vi "User Stop Event.vi"(0 "Stop":T2, 11 "Error in":errorcluster, 13 "Operations":T1) -> (4 "Stop Ref":refnum<user-event>, 15 "Error out":errorcluster)   [LabVIEW 2020, in "Data Communication Receiver.lvlib"]
doc: "User Event LV2 to stop the producer of the receiver."
uses:
  Data Communication Receiver.lvlib
  Typedefs/User Event Stop Data.ctl
  Typedefs/User event Operations.ctl
  Transmitter/Data Communication Transmitter.lvlib
panel:
  # "USER EVENT"
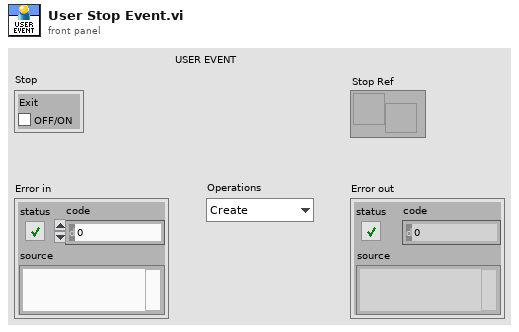
[diagram p1: front panel]
types:
  T1 = typedef "Data Communication Transmitter.lvlib/User event Operations.ctl" = enum16{"Create", "Generate", "Get Ref", "destroy"}
  T2 = typedef "Data Communication Receiver.lvlib/User Event Stop Data.ctl" = cluster{"Exit":bool}
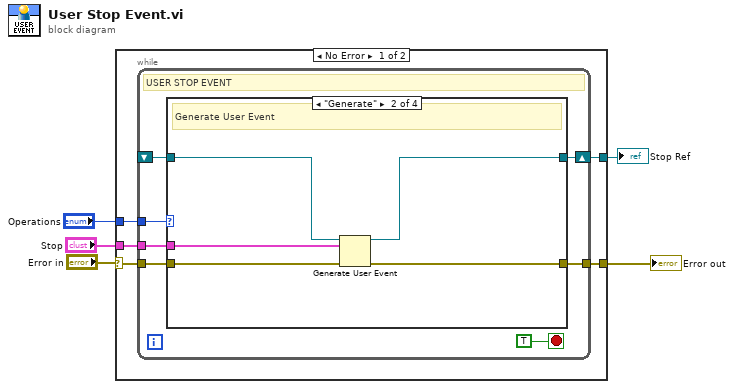
[diagram p0: block diagram]
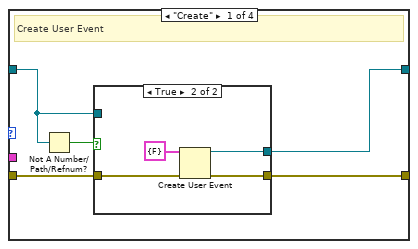
[diagram p2: hidden frame]
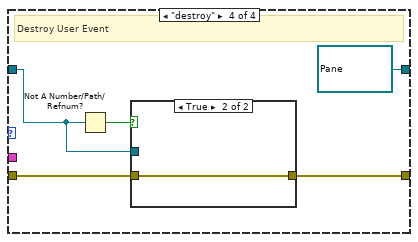
[diagram p5: hidden frame]
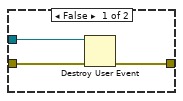
[diagram p6: hidden frame]
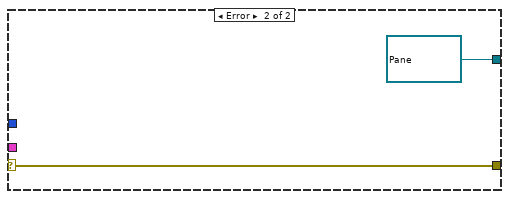
[diagram p7: hidden frame]
diagram:
  n1 = case shown="No Error" "Error in" {
    selector: "Error in" -> [w9 w46]
    tunnel: "Operations" -> [w10 _]
    tunnel: [w8 w46] -> w3
    tunnel: "Stop" -> [w7 _]
    tunnel: [w6 refnum<user-event> refnum ("Stop")] -> w1
    frame No Error {
      n2 = while {
        tunnel: w10 -> [w16]
        tunnel: w9 -> [w15]
        tunnel: [w14] -> w8
        shift-right: [w13] -> w6
        shift-left: _ -> [w12]
        tunnel: w7 -> [w11]
        stop <- TRUE stop-if-true
        # "USER STOP EVENT"
        n3 = case shown="\"Generate\"" w16 {
          tunnel: w15 -> [w22 w33 w35 w40]
          tunnel: [w21 w32 w35 w39] -> w14
          tunnel: [w20 w30 w34 refnum<user-event> refnum ("Stop")] -> w13
          tunnel: w12 -> [w18 w31 w34 w37]
          tunnel: w11 -> [_ w29 _ _]
          frame "Create" {
            # "Create User Event"
            n4 = Not A Number/Path/Refnum?(number/path/refnum=w18) -> (NaN/Path/Refnum?=w19:bool)
            n5 = case shown="True" w19 {
              tunnel: w22 -> [w24 w28]
              tunnel: [w24 w27] -> w21
              tunnel: [w23 w25] -> w20
              tunnel: w18 -> [w23 _]
              frame False {
              }
              frame True {
                n6 = Create User Event(user event datatype=T2 {"Exit"=FALSE} ("Stop"), error in=w28) -> (user event=w25:refnum<user-event>, error out=w27:errorcluster)
              }
            }
          }
          frame "Generate" {
            # "Generate User Event"
            n7 = Generate User Event(user event=w31, event data cluster=w29, error in=w33) -> (user event out=w30:refnum<user-event>, error out=w32:errorcluster)  [unwired: 1 in]
          }
          frame "Get Ref" {
            # "Get User Event Reference"
          }
          frame "destroy" {
            # "Destroy User Event"
            n8 = Not A Number/Path/Refnum?(number/path/refnum=w37) -> (NaN/Path/Refnum?=w38:bool)
            n9 = case shown="True" w38 {
              tunnel: w40 -> [w43 w44]
              tunnel: [w42 w44] -> w39
              tunnel: w37 -> [w41 _]
              frame False {
                n10 = Destroy User Event(user event=w41, error in=w43) -> (error out=w42:errorcluster)
              }
              frame True {
              }
            }
          }
        }
      }
    }
    frame Error {
    }
  }
  "Error out" <- w3
  "Stop Ref" <- w1
